vi "target.vi"   [LabVIEW 2020]
uses:
  <vilib>/rvi/interface/RandomDataEmulation/niFpgaRandomDataHandleErrors.vi
  dot_product_VIs/20_10_dot_product.vi
  <vilib>/rvi/DataTransferAndStorage/Container/XNode/niFpgaContainer.xnode
  <vilib>/rvi/interface/RandomDataEmulation/nirviRandomDataFpgaReadWriteTemplate.vi
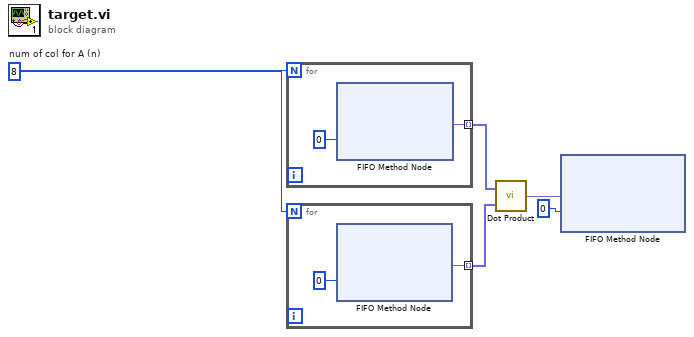
[diagram p0: block diagram]
diagram:
  w5 = 8  # num of col for A (n)
  n1 = for {
    N: w5 -> [_]
    tunnel: [w7] -> w3 mode=indexing
    n2 = xnode ("FIFO Method Node")("Timeout"=0) -> ("Element"=w7:fxp<+/-,20,10>)  [unwired: 1 in, 2 out]
  }
  n3 = for {
    N: w5 -> [_]
    tunnel: [w8] -> w2 mode=indexing
    n4 = xnode ("FIFO Method Node")("Timeout"=0) -> ("Element"=w8:fxp<+/-,20,10>)  [unwired: 1 in, 2 out]
  }
  n5 = call-poly "Dot Product.vi"("B"=w2, "A"=w3) -> ("c"=w1:fxp<+/-,20,10>)
  n6 = xnode ("FIFO Method Node")("Element"=w1, "Timeout"=0) -> ()  [unwired: 1 in, 2 out]
